vi "Read Temperature.vi"(8 "error in (no error)":errorcluster, 11 "Bronkhorst Settings in":T1={"VISA resource name"="", "Simulated?"=FALSE, "Smoothing Steps"=1} {"Smoothing Steps" min=1 step=1}) -> (0 "error out":errorcluster, 1 "Connection Error":bool, 2 "Temp (C)":sgl, 3 "Bronkhorst Settings out":T1={"VISA resource name"="", "Simulated?"=FALSE, "Smoothing Steps"=1} {"Smoothing Steps" min=1 step=1})   [LabVIEW 2018, in "Bronkhorst M13 Flow Meter.lvlib"]
uses:
  Bronkhorst M13 Flow Meter.lvlib
  Settings Cluster.ctl
  <vilib>/regexp/Match Regular Expression.xnode
  <vilib>/ptbypt/NI_PtbyPt.lvlib
panel:
  out "x+1":u32
  out "read buffer 2":string
  out "submatch 1":string
  out "whole match":string
  out "read buffer":string
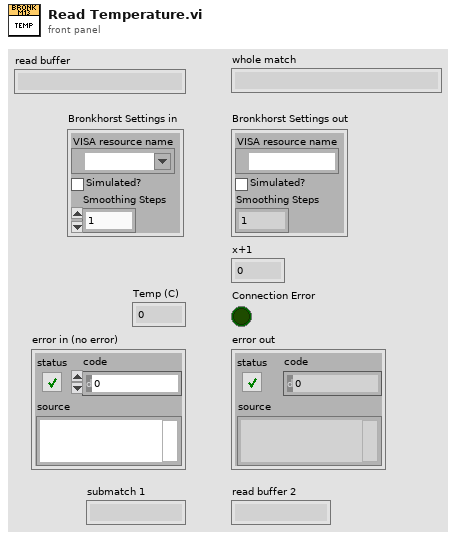
[diagram p1: front panel]
types:
  T1 = typedef "Bronkhorst M13 Flow Meter.lvlib/Settings Cluster.ctl" = cluster{"VISA resource name":refnum<visa-resource-name>, "Simulated?":bool, "Smoothing Steps":i32}
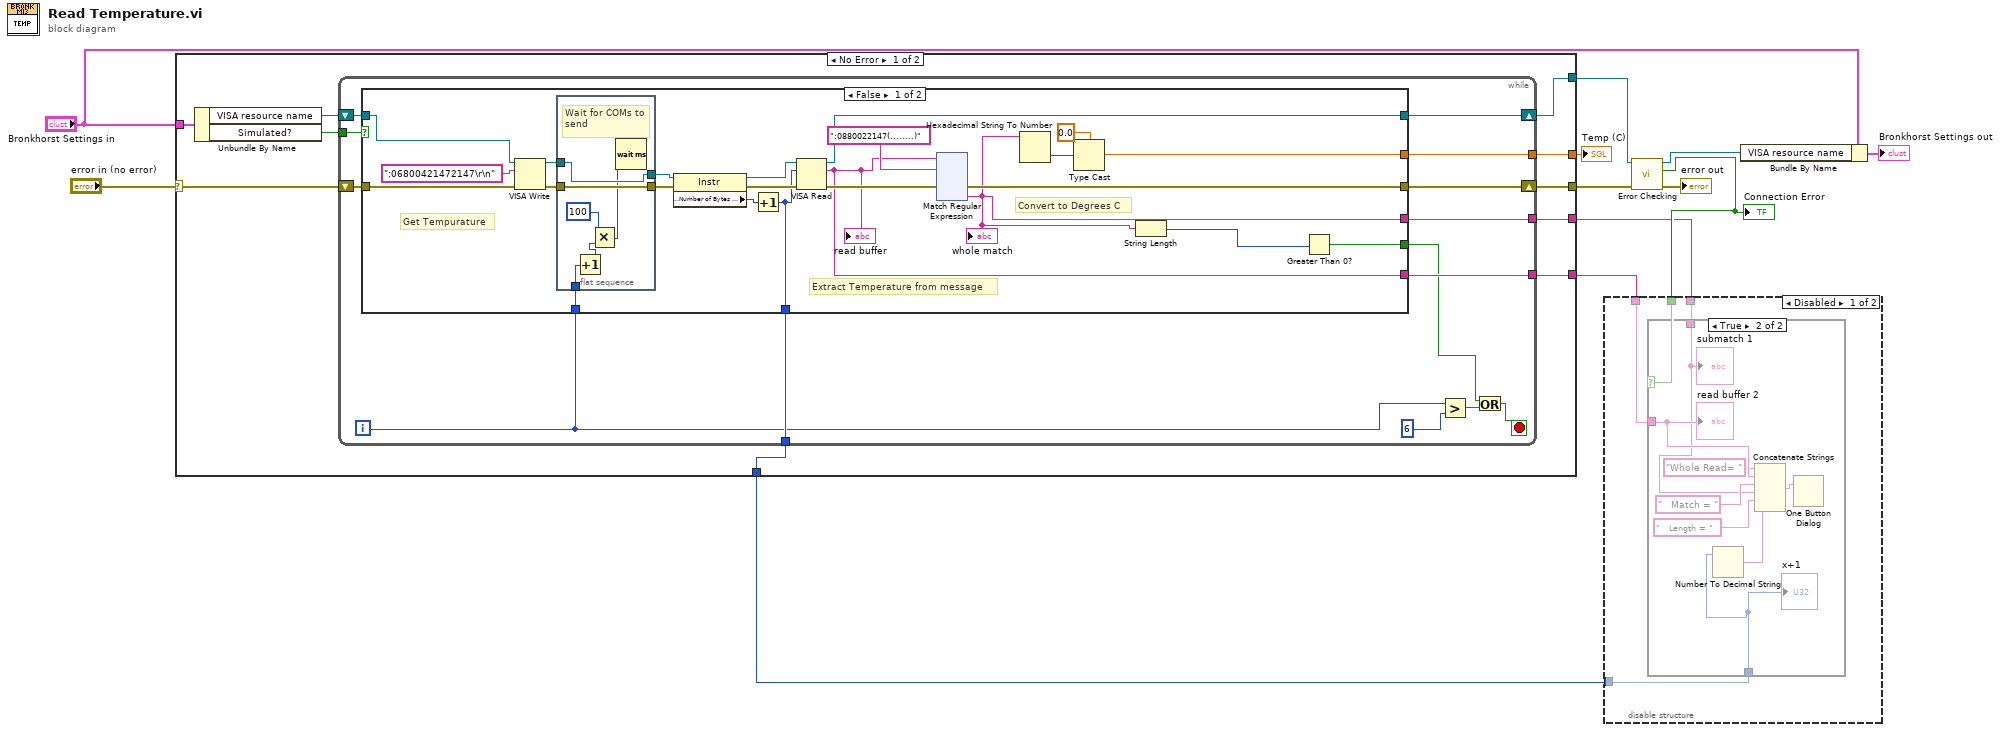
[diagram p0: block diagram]
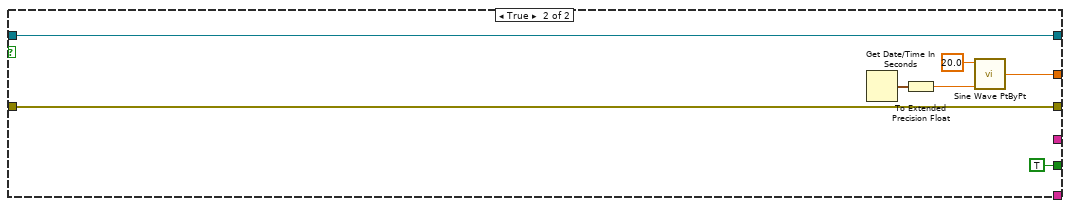
[diagram p4: hidden frame]
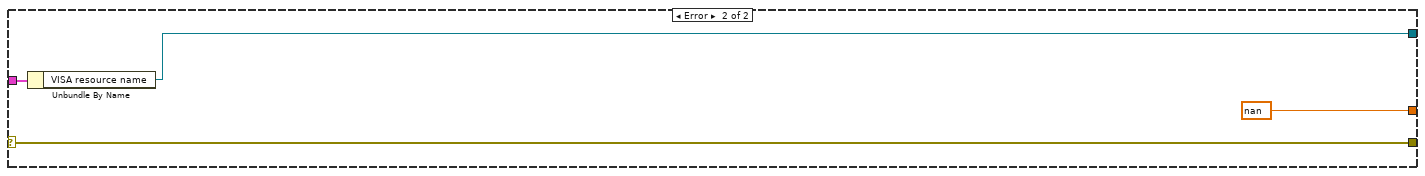
[diagram p5: hidden frame]
diagram:
  n1 = case shown="No Error" "error in (no error)" {
    selector: "error in (no error)" -> [w21 w192]
    tunnel: [w20 w192] -> w7
    tunnel: "Bronkhorst Settings in" -> [w19 w191]
    tunnel: [w17 w190] -> w9
    tunnel: [w16 nan ("sine wave")] -> w5
    tunnel: [w15 _] -> w3
    tunnel: [w14 _] -> w2
    tunnel: [w13 _] -> w1
    frame No Error {
      n2 = Unbundle By Name(w19) -> ("VISA resource name"=w18:refnum<visa-resource-name>, "Simulated?"=w22:bool)
      n3 = while {
        tunnel: w22 -> [w36]
        tunnel: [w31] -> w16
        tunnel: [w30] -> w15
        tunnel: [w29] -> w14
        tunnel: [w28] -> w13
        shift-right: [w34] -> w20
        shift-left: w21 -> [w35]
        shift-right: [w32] -> w17
        shift-left: w18 -> [w33]
        i -> [w23]
        stop <- w24 stop-if-true
        n4 = case shown="False" w36 {
          tunnel: [w43 w188] -> w34
          tunnel: w35 -> [w51 w188]
          tunnel: [w49 w184] -> w32
          tunnel: w33 -> [w52 w184]
          tunnel: [w46 w183] -> w31
          tunnel: [w40 _] -> w30
          tunnel: [w42 _] -> w29
          tunnel: [w41 _] -> w28
          tunnel: [w37 TRUE] -> w25
          tunnel: w23 -> [w39 _]
          frame False {
            # "Extract Temperature from message"
            # "Get Tempurature"
            # "Convert to Degrees C"
            n5 = VISA Write(VISA resource name=w52, write buffer=":06800421472147\r\n" ("Command"), error in (no error)=w51) -> (VISA resource name out=w56:refnum<visa-resource-name>, error out=w54:errorcluster)  [unwired: 1 out]
            n6 = flat-sequence {
              tunnel: [w181] -> w55
              tunnel: w56 -> [w181]
              tunnel: [w180] -> w53
              tunnel: w54 -> [w180]
              tunnel: w39 -> [w177]
              frame #0 {
                # "Wait for COMs to send"
                n7 = Increment(x=w177) -> (x+1=w176:i32)
                n8 = Multiply(x=u32 100 ("milliseconds to wait"), y=w176) -> (x*y=w178:u32)
                n9 = Wait (ms)(milliseconds to wait=w178) -> ()  [unwired: 1 out]
              }
            }
            n10 = property class="Instr"(reference=w55, error in=w53) -> (reference out=w58:refnum<visa-resource-name>, error out=w57:errorcluster, "Serial Settings:Number of Bytes at Serial Port"=w50:u32)
            n11 = Increment(x=w50) -> (x+1=w41:u32)
            n12 = VISA Read(VISA resource name=w58, byte count=w41, error in (no error)=w57) -> (VISA resource name out=w49:refnum<visa-resource-name>, read buffer=w42:string, error out=w44:errorcluster)  [unwired: 1 out]
            "read buffer" <- w42
            n13 = xnode "Match Regular Expression"("input string"=w42, "regular expression"=":0880022147(........)" ("Regular Expression for Extracting Weight"), "error in"=w44) -> ("error out"=w43:errorcluster, "submatch 1"=w40:string)  [unwired: 3 in, 4 out]
            "whole match" <- w40
            n14 = Hexadecimal String To Number(string=w40) -> (number=w47:u32)  [unwired: 2 in, 1 out]
            n15 = Type Cast(type=sgl 0.0, x=w47) -> (*(type *) &x=w46:sgl)
            n16 = String Length(string=w40) -> (length=w38:i32)
            n17 = Greater Than 0?(x=w38) -> (x > 0?=w37:bool)
          }
          frame True {
            n18 = Get Date/Time In Seconds() -> (seconds since 1Jan1904=w187:timestamp)
            n19 = To Extended Precision Float(1:w187) -> (0:w186:ext)
            n20 = call <vilib>:"Sine Wave PtByPt.vi"("time"=w186, "amplitude"=20.0) -> ("sine wave"=w183:dbl)  [unwired: 2 in]
          }
        }
        n21 = Greater?(x=w23, y=6) -> (0:w26:bool)
        n22 = Or(x=w25, y=w26) -> (x .or. y?=w24:bool)
      }
    }
    frame Error {
      n23 = Unbundle By Name(w191) -> ("VISA resource name"=w190:refnum<visa-resource-name>)
    }
  }
  "Temp (C)" <- w5
  n24 = call "Error Checking.vi"("error in (no error)"=w7, "VISA resource name"=w9) -> ("error out"=→"error out":errorcluster, "Connection Error"=w4:bool, "VISA resource name"=w8:refnum<visa-resource-name>)  [unwired: 7 in]
  "Connection Error" <- w4
  n25 = disable-structure shown="Disabled" {
    disable-tunnel: w4 -> [w196 _]
    disable-tunnel: w3 -> [w195 _]
    disable-tunnel: w2 -> [w194 _]
    disable-tunnel: w1 -> [w193 _]
    frame Disabled {
      n26 = case shown="True" w196 {
        tunnel: w195 -> [_ w200]
        tunnel: w194 -> [_ w203]
        tunnel: w193 -> [_ w198]
        frame False {
        }
        frame True {
          n27 = Number To Decimal String(number=w198) -> (decimal integer string=w197:string)  [unwired: 1 in]
          n28 = Concatenate Strings("Whole Read= " ("string"), w203, "   Match = " ("string"), w200, "   Length = " ("string"), w197) -> (w204:string)
          n29 = One Button Dialog(message=w204) -> ()  [unwired: 1 in, 1 out]
          "submatch 1" <- w200
          "read buffer 2" <- w203
          "x+1" <- w198
        }
      }
    }
    frame Enabled {
    }
  }
  n30 = Bundle By Name(cluster="Bronkhorst Settings in", "VISA resource name"=w8) -> (→"Bronkhorst Settings out":T1)
